vi "Status Monitor (Multi Unit - Fast Parallel Read).vi"(11 "INI Array":path[](array[path])) -> (0 "error out":errorcluster)   [LabVIEW 2017, in "Status Monitor Library.lvlib"]
uses:
  Status Monitor Library.lvlib
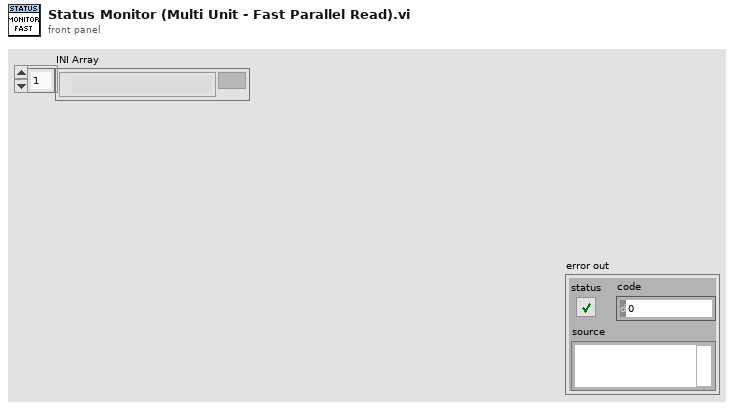
[diagram p1: front panel]
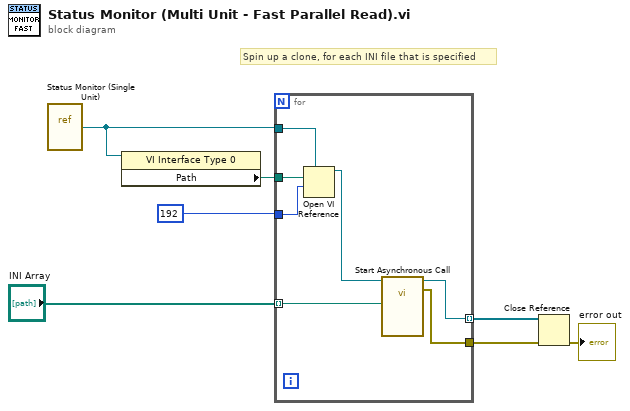
[diagram p0: block diagram]
diagram:
  # "Spin up a clone, for each INI file that is specified"
  n1 = vi-ref "Status Monitor (Single Unit).vi"() -> (w3:refnum<vi>)
  n2 = property class="VI Interface Type 0"(reference=w3) -> ("Path"=w2:path)  [unwired: 1 in, 2 out]
  n3 = for {
    tunnel: "INI Array" -> [w14] mode=indexing
    tunnel: w3 -> [w13]
    tunnel: w2 -> [w12]
    tunnel: 192 ("options") -> [w11]
    tunnel: [w9] -> w5 mode=indexing
    tunnel: [w8] -> w4
    n4 = Open VI Reference(type specifier VI Refnum (for type only)=w13, vi path=w12, options=w11) -> (vi reference=w10:refnum<vi>)  [unwired: 3 in, 1 out]
    n5 = call-by-ref "Start Asynchronous Call"(reference=w10, "configuration file path"=w14) -> (reference out=w9:refnum<vi>, error out=w8:errorcluster)  [unwired: 12 in]
  }
  n6 = Close Reference(reference=w5, error in (no error)=w4) -> (error out=→"error out":errorcluster)
